vi "SQL_table_test_selectbyid.vi"(11 "testId":string) -> (3 "tester":string)   [LabVIEW 2014]
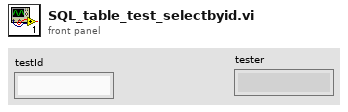
[diagram p1: front panel]
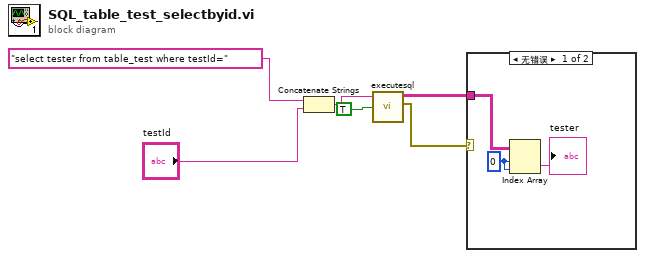
[diagram p0: block diagram]
diagram:
  n1 = Concatenate Strings("select tester from table_test where testId=" ("Command Text"), "testId") -> (w5:string)
  n2 = call "executesql.vi"("Return Data (T)"=TRUE, "Command Text"=w5) -> ("error out"=w3:errorcluster, "Data"=w2:string[][])  [unwired: 5 in]
  n3 = case shown="无错误" w3 {
    tunnel: w2 -> [w9 _]
    frame No Error {
      w8 = 0 ("索引 (行)")
      n4 = Index Array(array=w9, index (row)=w8, index (col)=w8) -> (element=→"tester":string)
    }
    frame Error {
    }
  }
